vi "TSM Relays to Relay Sessions.vi"(0 "TSM Context":T2, 5 "Relays":tag[](array[tag]), 11 "error in (no error)":errorcluster) -> (4 "TSM Relay Out":T1, 15 "error out":errorcluster)   [LabVIEW 2019]
doc: "Populates the Relay cluster for the selected relays."
uses:
  <vilib>/NI_TestStand_SemiconductorModule/NI_TestStand_Semiconductor_Module.lvlibp/PinMap/General/SemiconductorModuleContext.ctl
  TSM Relay.ctl
  <vilib>/NI_TestStand_SemiconductorModule/NI_TestStand_Semiconductor_Module.lvlibp
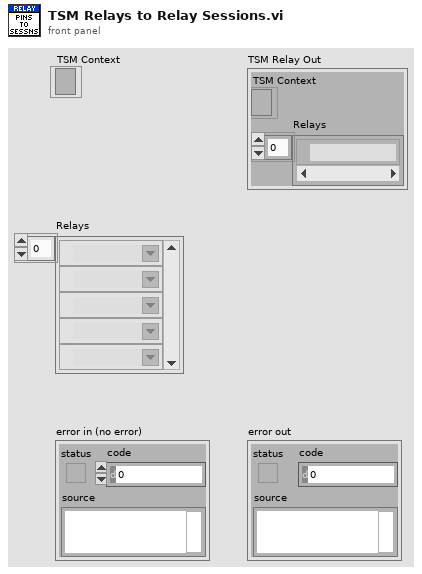
[diagram p1: front panel]
types:
  T1 = typedef "TSM Relay.ctl" = cluster{"TSM Context":T2, "Relays":tag[]}
  T2 = typedef "NI_TestStand_Semiconductor_Module.lvlibp/SemiconductorModuleContext.ctl" = refnum<k7>
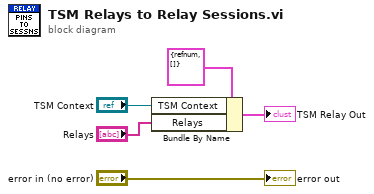
[diagram p0: block diagram]
diagram:
  n1 = Bundle By Name(cluster=T1 {"TSM Context"=refnum, "Relays"=[]} ("Relay TSM"), "TSM Context"="TSM Context", "Relays"="Relays") -> (→"TSM Relay Out":T1)
  "error out" <- "error in (no error)"
